vi "ReadSqlite3_handle.vi"(8 "error in (no error)":errorcluster, 11 "object in":refnum<class "SQLiteConnection.lvclass">) -> (0 "error out":errorcluster, 2 "sqlite3_handle":u64, 3 "object out":refnum<class "SQLiteConnection.lvclass">)   [LabVIEW 2019, in "SQLiteConnection.lvclass"]
uses:
  SQLiteConnection.lvclass
  SQLiteConnection.lvclass/SQLiteConnection.ctl
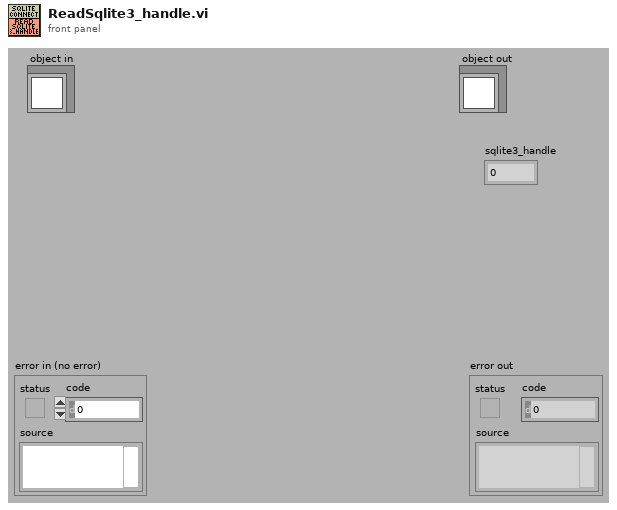
[diagram p1: front panel]
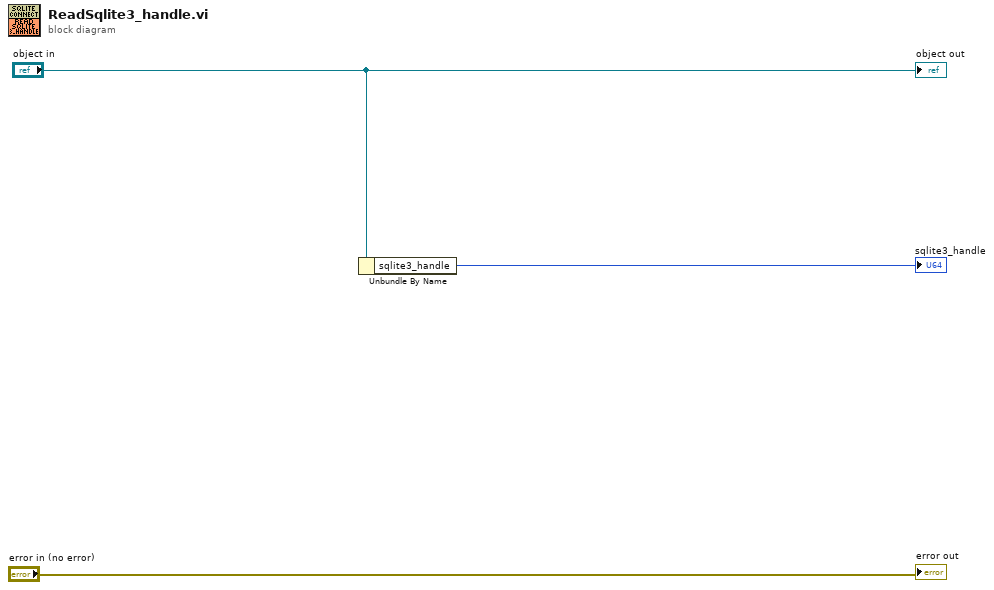
[diagram p0: block diagram]
diagram:
  n1 = Unbundle By Name("object in") -> ("sqlite3_handle"=→"sqlite3_handle":u64)
  "error out" <- "error in (no error)"
  "object out" <- "object in"
